vi "Start Collect.vi"(7 "Lasers ON?":bool, 8 "error in (no error)":errorcluster, 9 "Sample Data notifier":refnum<notifier>, 10 "data value reference":refnum<data-value>, 11 "Move Length":i32) -> (0 "error out":errorcluster, 1 "timed out?":bool, 3 "Start Collect (Reply Payload)":T1)   [LabVIEW 2015, in "Collect Data Mgr.lvlib"]
doc: "_____\nCreated using Delacor QMH Event Scripter 2.1.0.3."
uses:
  Collect Data Mgr.lvlib
  Start Collect (Reply Payload)--cluster.ctl
  Start Collect Argument--cluster.ctl
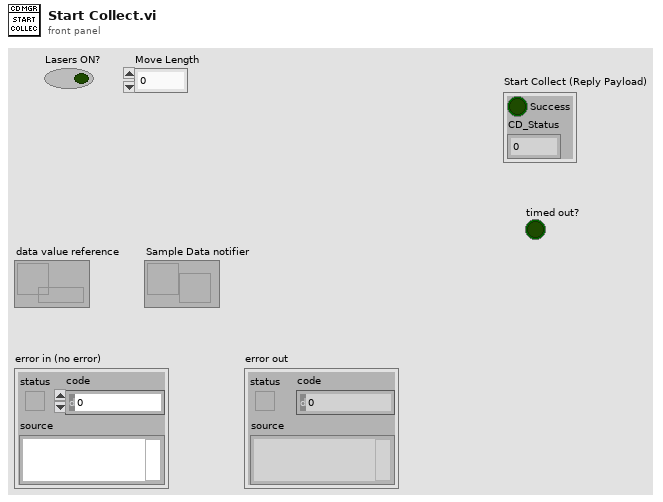
[diagram p1: front panel]
types:
  T1 = typedef "Collect Data Mgr.lvlib/Start Collect (Reply Payload)--cluster.ctl" = cluster{"Success":bool, "CD_Status":u8}
  T2 = typedef "Collect Data Mgr.lvlib/Start Collect Argument--cluster.ctl" = cluster{"Lasers ON?":bool, "Move Length":i32, "Sample Data notifier":refnum<notifier>, "data value reference":refnum<data-value>, "Wait Notifier":refnum<notifier>}
  T3 = typedef "Collect Data Mgr.lvlib/Request Events--cluster.ctl" = cluster{"Stop Module":refnum<user-event>, "Show Panel":refnum<user-event>, "Hide Panel":refnum<user-event>, "Get Module Execution Status":refnum<user-event>, "Show Diagram":refnum<user-event>, "Start Collect":refnum<user-event>, "Stop Collect":refnum<user-event>}
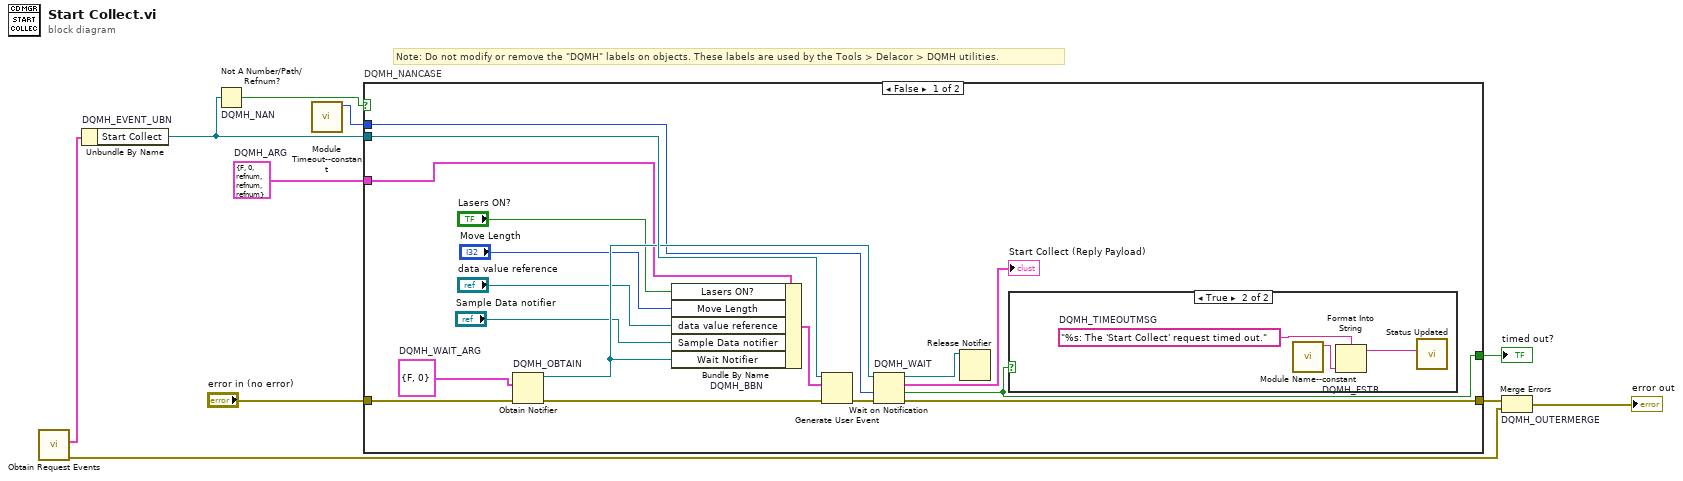
[diagram p0: block diagram]
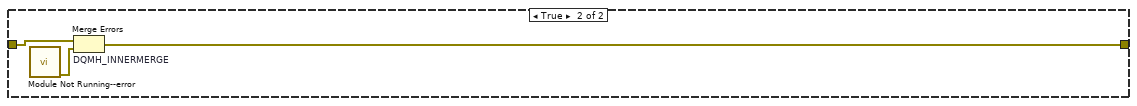
[diagram p3: hidden frame]
diagram:
  w4 = T2 {"Lasers ON?"=FALSE, "Move Length"=0, "Sample Data notifier"=refnum, "data value reference"=refnum, "Wait Notifier"=refnum}  # DQMH_ARG
  # "Note: Do not modify or remove the \"DQMH\" labels on objects. These labels are used by the Tools > Delacor > DQMH utilities."
  n1 = call "Obtain Request Events.vi"() -> ("error out"=w2:errorcluster, "Probe Mgr Request Events"=w1:T3)  [unwired: 10 in]
  n2 = Unbundle By Name "DQMH_EVENT_UBN"(w1) -> ("Start Collect"=w8:refnum<user-event>)
  n3 = Not A Number/Path/Refnum? "DQMH_NAN"(number/path/refnum=w8) -> (NaN/Path/Refnum?=w7:bool)
  n4 = call "Module Timeout--constant.vi"() -> ("Module Timeout"=w3:i32)  [unwired: 11 in]
  n5 = case "DQMH_NANCASE" shown="False" w7 {
    tunnel: "error in (no error)" -> [w27 w33]
    tunnel: w8 -> [w25 _]
    tunnel: [w21 w32] -> w5
    tunnel: [w18 _] -> w6
    tunnel: w4 -> [w17 _]
    tunnel: w3 -> [w16 _]
    frame False {
      w22 = T1 {"Success"=FALSE, "CD_Status"=0}  # DQMH_WAIT_ARG
      n6 = Obtain Notifier "DQMH_OBTAIN"(notification data type=w22, error in (no error)=w27) -> (notifier out=w20:refnum<notifier>, error out=w23:errorcluster)  [unwired: 2 in, 1 out]
      n7 = Bundle By Name "DQMH_BBN"(cluster=w17, "Lasers ON?"="Lasers ON?", "Move Length"="Move Length", "data value reference"="data value reference", "Sample Data notifier"="Sample Data notifier", "Wait Notifier"=w20) -> (w24:T2)
      n8 = Generate User Event(user event=w25, event data cluster=w24, error in=w23) -> (error out=w26:errorcluster)  [unwired: 1 in, 1 out]
      n9 = Wait on Notification "DQMH_WAIT"(notifier=w20, timeout in ms (-1)=w16, error in (no error)=w26) -> (notifier out=w19:refnum<notifier>, notification=→"Start Collect (Reply Payload)":T1, timed out?=w18:bool, error out=w21:errorcluster)  [unwired: 1 in]
      n10 = Release Notifier(notifier=w19) -> ()  [unwired: 2 in, 3 out]
      n11 = case shown="True" w18 {
        frame False {
        }
        frame True {
          w30 = "%s: The 'Start Collect' request timed out."  # DQMH_TIMEOUTMSG
          n12 = call "Module Name--constant.vi"() -> ("Module Name"=w29:string)  [unwired: 11 in]
          n13 = Format Into String "DQMH_FSTR"(format string=w30, w29) -> (resulting string=w28:string)  [unwired: 2 in, 1 out]
          n14 = call "Status Updated.vi"("Status"=w28) -> ()  [unwired: 10 in, 1 out]
        }
      }
    }
    frame True {
      n15 = call "Module Not Running--error.vi"() -> ("error out"=w31:errorcluster)  [unwired: 11 in]
      n16 = Merge Errors "DQMH_INNERMERGE"(w33, w31) -> (w32:errorcluster)
    }
  }
  "timed out?" <- w6
  n17 = Merge Errors "DQMH_OUTERMERGE"(w5, w2) -> (→"error out":errorcluster)
